vi "MeasurementServer_SetResponse_FourProbeMeasurement.vi"(0 "gRPCid":T4, 1 "FourProbeResponse":T1, 3 "error in (no error)":errorcluster) -> (10 "error out":errorcluster)   [LabVIEW 2019, in "labview-grpc-measurement-server.lvlib"]
uses:
  labview-grpc-measurement-server.lvlib
  MeasurementServer_gRPCid.ctl
  MeasurementServer_FourProbeResponse.ctl
  MeasurementServer_FourProbeRawData.ctl
  MeasurementServer_ErrorOutData.ctl
  home/lvuser/liblabview_measurement_server.so
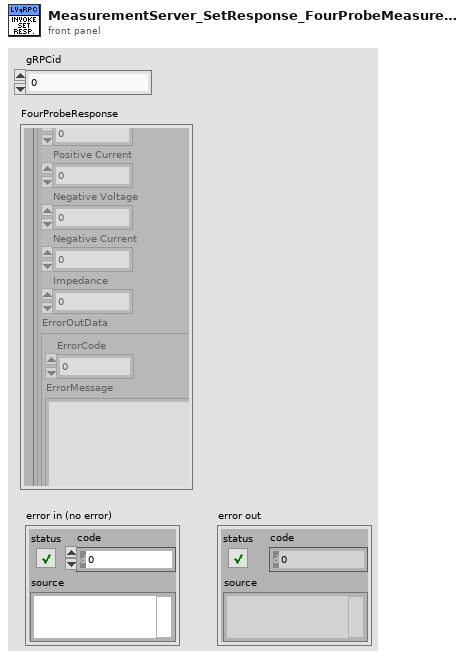
[diagram p1: front panel]
types:
  T1 = typedef "labview-grpc-measurement-server.lvlib/MeasurementServer_FourProbeResponse.ctl" = cluster{"Results":T2[]}
  T2 = typedef "labview-grpc-measurement-server.lvlib/MeasurementServer_FourProbeRawData.ctl" = cluster{"Positive Voltage":dbl, "Positive Current":dbl, "Negative Voltage":dbl, "Negative Current":dbl, "Impedance":dbl, "ErrorOutData":T3}
  T3 = typedef "labview-grpc-measurement-server.lvlib/MeasurementServer_ErrorOutData.ctl" = cluster{"ErrorCode":i32, "ErrorMessage":string}
  T4 = typedef "labview-grpc-measurement-server.lvlib/MeasurementServer_gRPCid.ctl" = u64
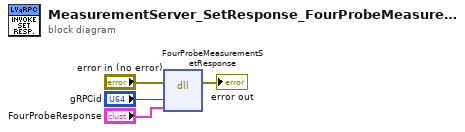
[diagram p0: block diagram]
diagram:
  n1 = dll-call lib="home/lvuser/liblabview_measurement_server.so" fn="FourProbeMeasurementSetResponse"(error in="error in (no error)", "id"="gRPCid", "data"="FourProbeResponse") -> (error out=→"error out":errorcluster)  [unwired: 5 in, 1 out]
